vi "main_link.vi"() -> ()   [LabVIEW 2023]
uses:
  <vilib>/Math Plots/3D Math Plots/3D Scatter/3D Scatter XCtrl/3D Scatter.xctl
  HoloTrackerLib/holoTracker.lvlib
  subVis/referencesLINKBtns.ctl
  HoloTrackerLib/dataLink.ctl
  <vilib>/Utility/miscctls.llb/LVMinMaxIncTypeDef.ctl
  subVis/defValuesLink.ctl
  <vilib>/Math Plots/3D Math Plots/3D Scatter/3D Scatter Datatype/3D Scatter Datatype.lvclass
  <vilib>/Math Plots/3D Math Plots/3D Scatter/3D Scatter Datatype/Public/Plot Helper (Vector).vi
  <vilib>/Python/Open Venv Python Session.vi
panel:
  out "Status":string
  in  "Tab Control":enum32{"PATH", "ACTIONS"}(tab)=enum."ACTIONS"
  in  "HoloPath":path caption="feature localisation file path"
  in  "PythonVer":string="3.10" caption="Python version"
  in  "Python/Environnement\npath":path
  in  "step":u16 max=1001 step=1
  in  "history length":u16 max=1001 step=1
  in  "min length":i32
  in  "searchRange":T1={"x_range(m)"=1e-06, "y_range(m)"=1e-06, "z__range(m)"=1e-06}
  in  "memory":i32
  in  "Feature hologram":u16 max=1001 step=1
  in  "SAVE":bool
  out "Total trajectories":u16=95 max=200
  in  "trajectory":u16 max=0
  in  "LINK":bool
  in  "OpenFile":bool
  in  "EXIT":bool
  out "Total holograms":u16=95 max=200
  in  "Play":bool
  in  "CancelPlay":bool
  out "3D Scatter":refnum<class "3D Plot Datatype.lvclass">[](xcontrol)
  # "Link parameters"
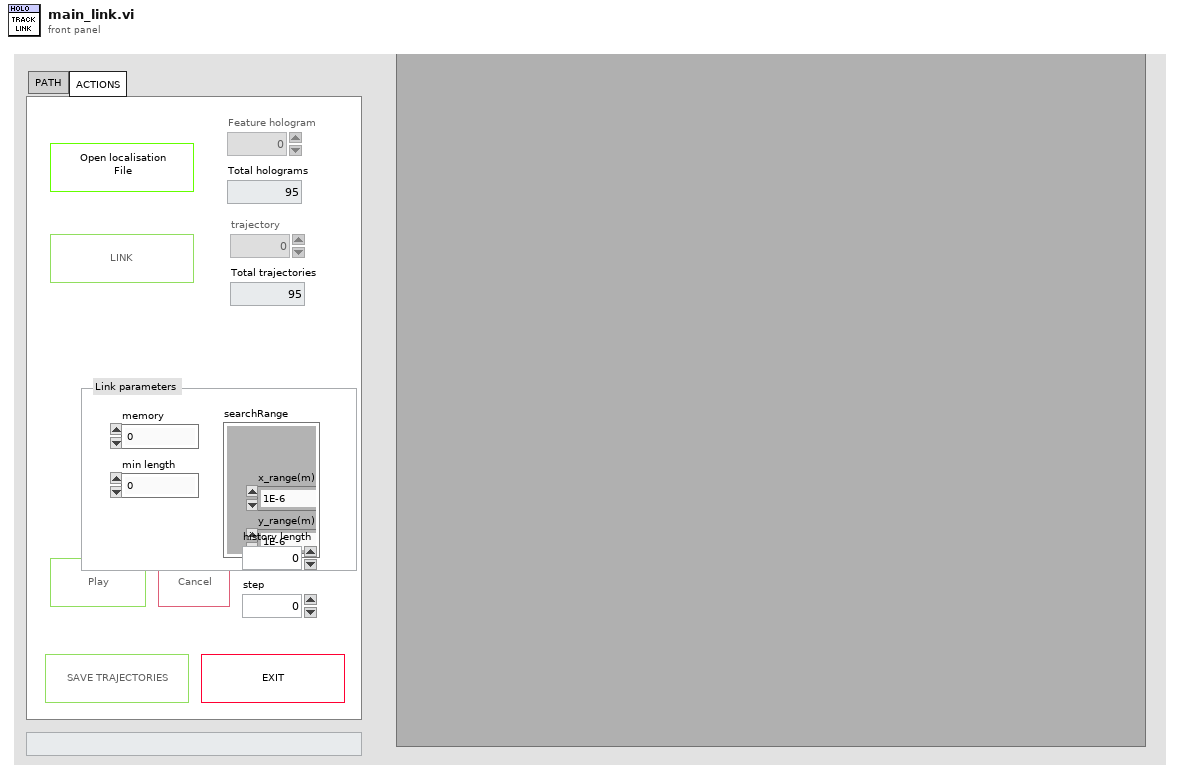
[diagram p1: front panel]
types:
  T1 = cluster{"x_range(m)":dbl, "y_range(m)":dbl, "z__range(m)":dbl}
  T2 = typedef "referencesLINKBtns.ctl" = cluster{"PythonVer":refnum<vi>, "Python/Environnement\npath":refnum<vi>, "HoloPath":refnum<vi>, "HoloDir":refnum<vi>, "Holo parameters":refnum<vi>, "Remove mean Hologram":refnum<vi>, "propagation":refnum<vi>, "Fourier BP filter (pix)":refnum<vi>, "Focus":refnum<vi>, "Batch thresold ":refnum<vi>, "CCL parameters":refnum<vi>, "testMode":refnum<vi>, "exitTestMode":refnum<vi>, "BATCH":refnum<vi>, "CANCEL_BATCH":refnum<vi>, "EXIT":refnum<vi>, "Plane number":refnum<vi>, "Display":refnum<vi>}
  T3 = enum8{"Enabled", "Disabled", "Disabled and Grayed Out"}
  T4 = typedef "dataLink.ctl" = cluster{"PythonSession":refnum<k35>, "Localisations":sgl[][]}
  T5 = enum16{"SESSION CLOSED", "WAIT", "TEST WAIT", "TEST IN PROGESS", "BATCH IN PROGRESS"}
  T6 = typedef "LVMinMaxIncTypeDef.ctl" = cluster{"Minimum":dbl, "Maximum":dbl, "Increment":dbl}
  T7 = cluster{"frame_max":i32, "AllTrajectories":dbl[][]}
  T8 = typedef "defValuesLink.ctl" = cluster{"PythonVer":string, "Python/Environnement\npath":path, "HoloPath":path, "memory":i32, "min length":i32, "searchRange":cluster{"x_range(m)":dbl, "y_range(m)":dbl, "z__range(m)":dbl}}
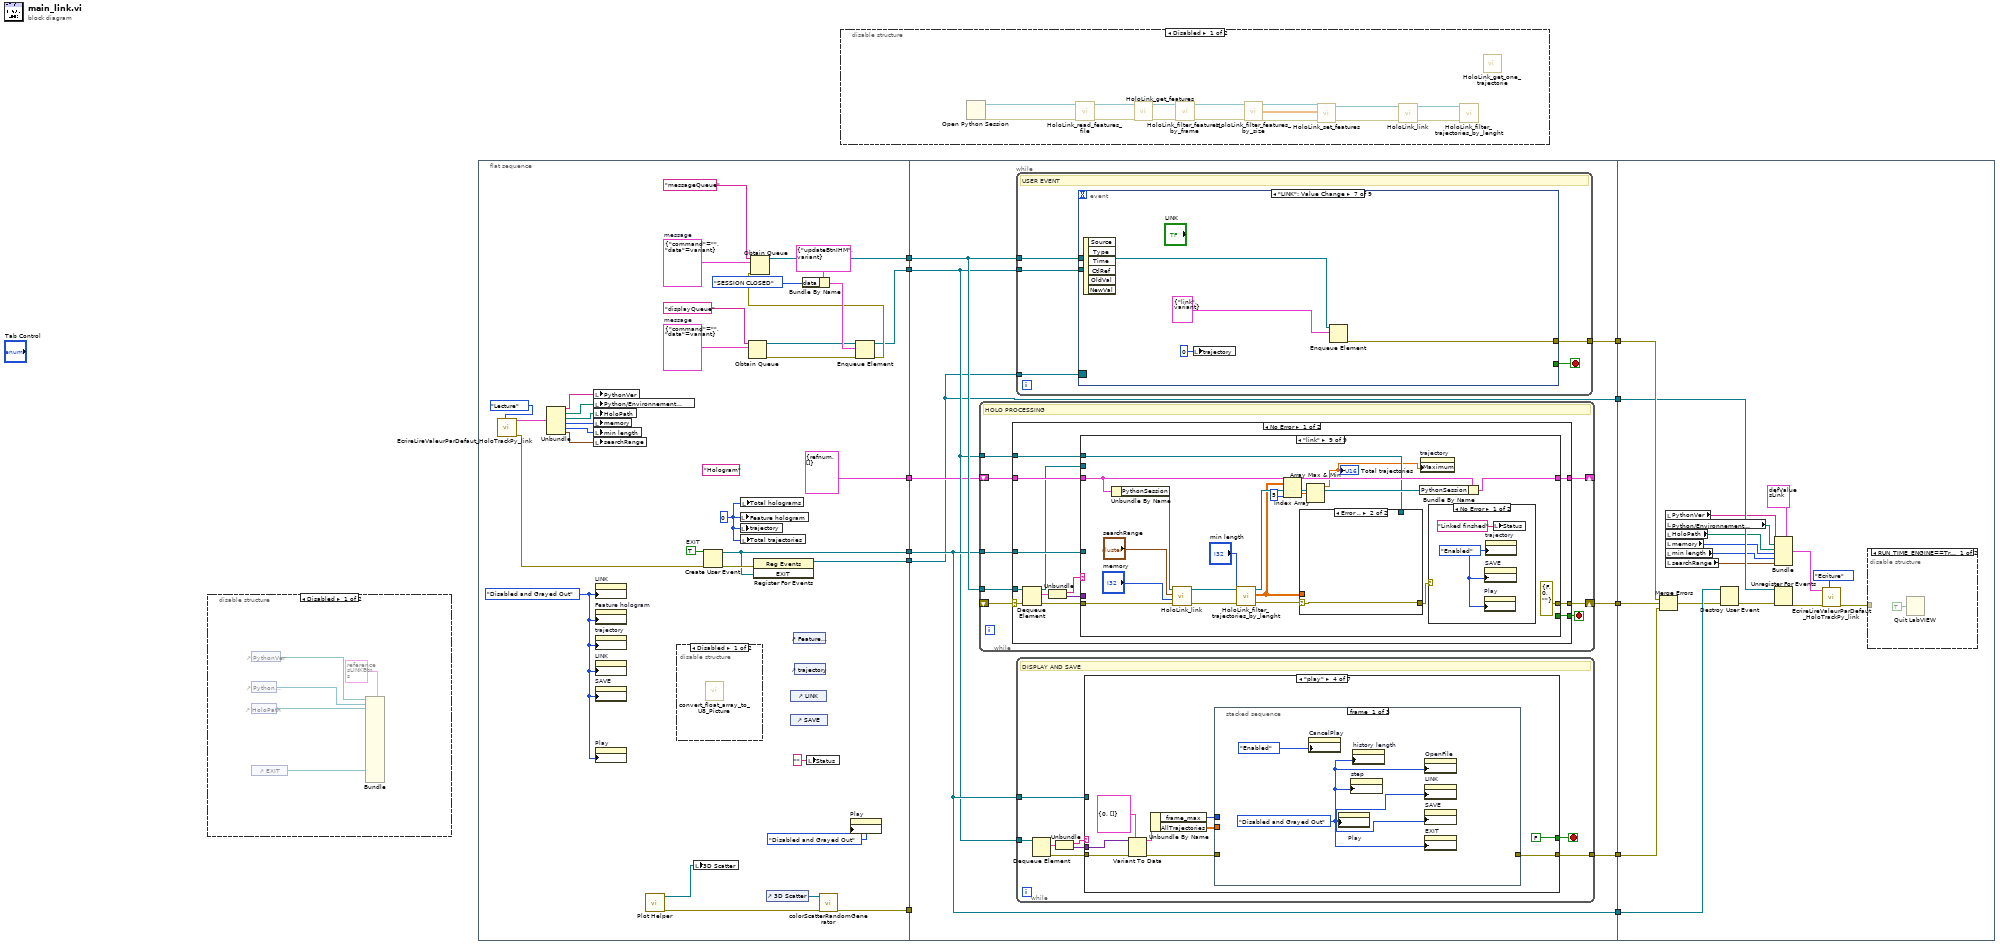
[diagram p0: block diagram]
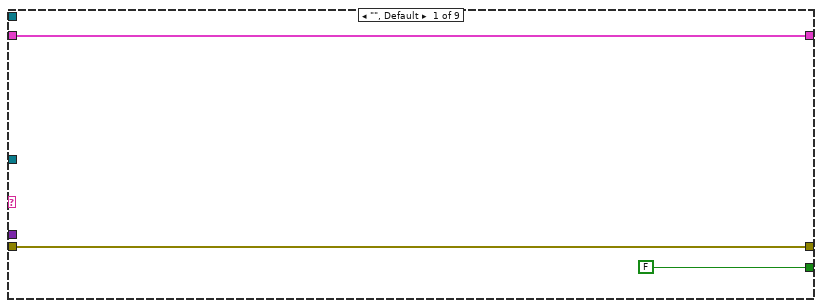
[diagram p5: hidden frame]
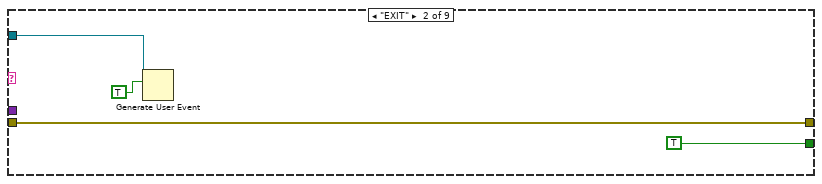
[diagram p6: hidden frame]
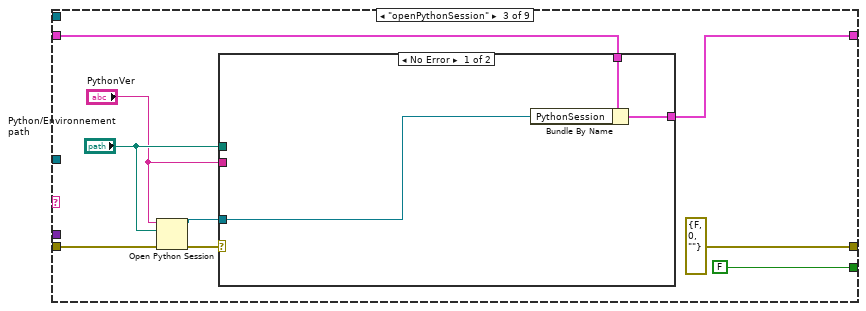
[diagram p7: hidden frame]
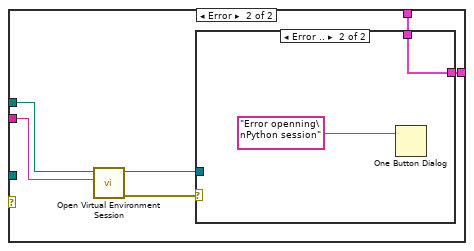
[diagram p8: hidden frame]
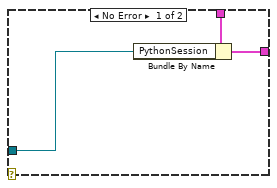
[diagram p9: hidden frame]
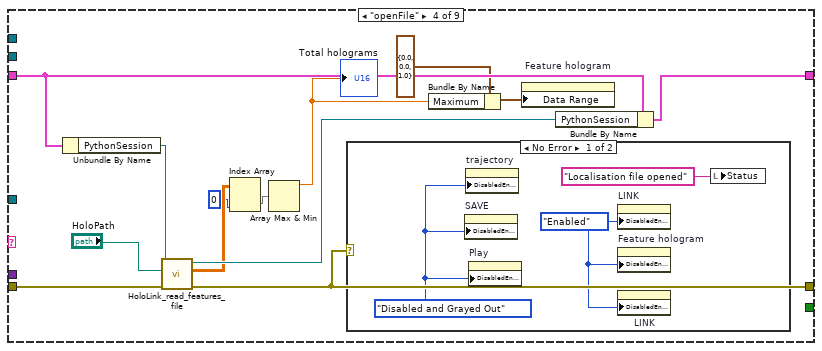
[diagram p10: hidden frame]
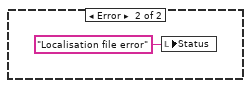
[diagram p11: hidden frame]
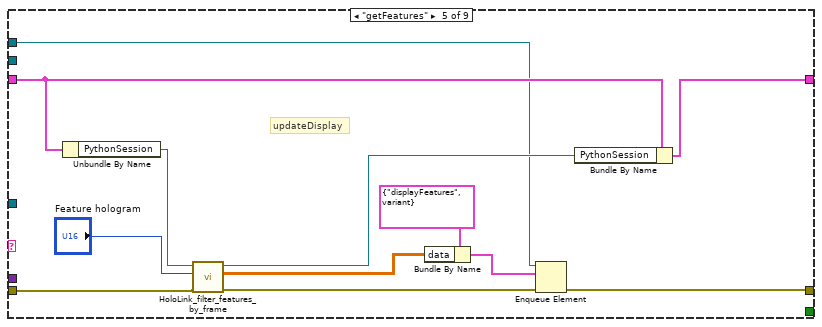
[diagram p12: hidden frame]
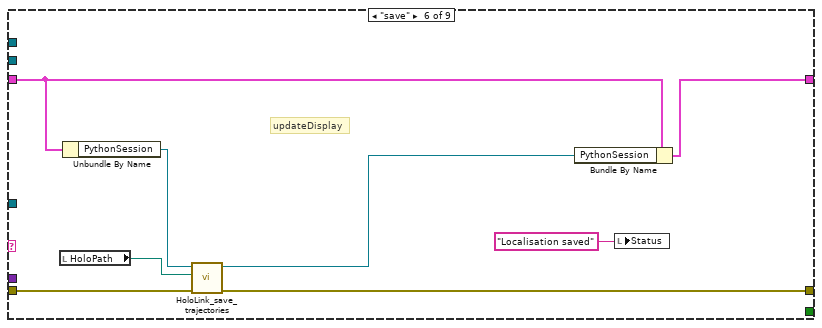
[diagram p13: hidden frame]
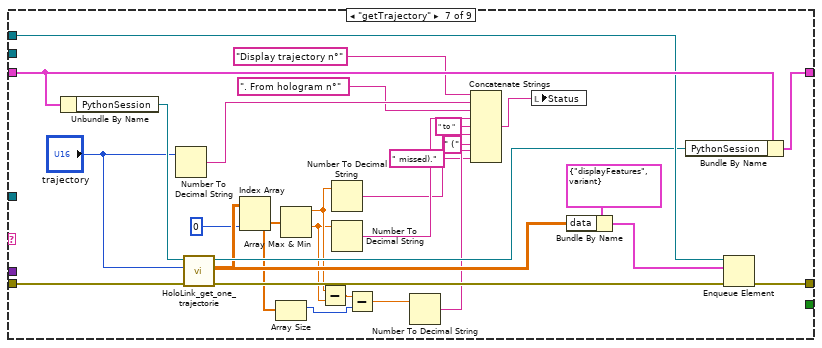
[diagram p14: hidden frame]
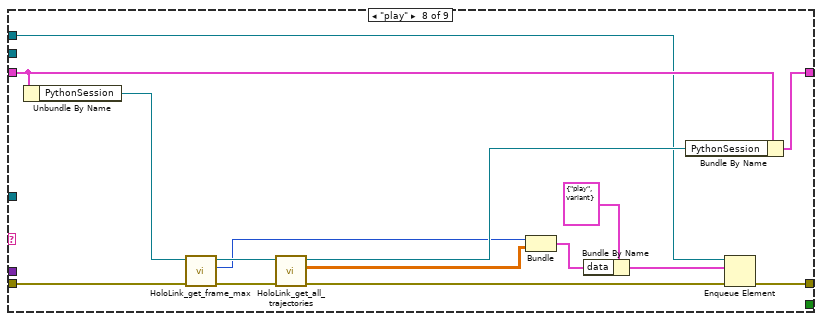
[diagram p15: hidden frame]
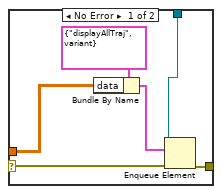
[diagram p16: hidden frame]
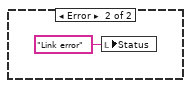
[diagram p17: hidden frame]
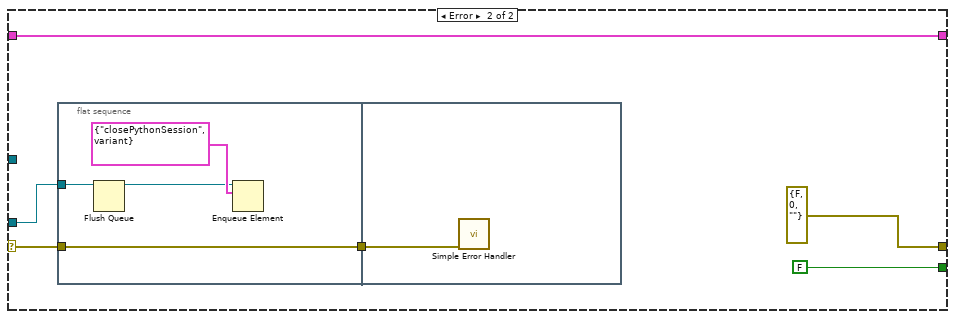
[diagram p18: hidden frame]
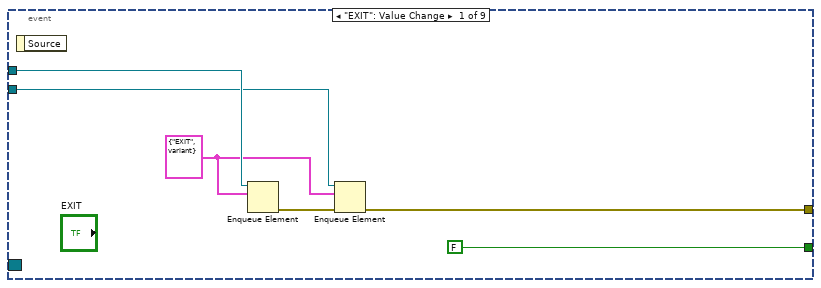
[diagram p19: hidden frame]
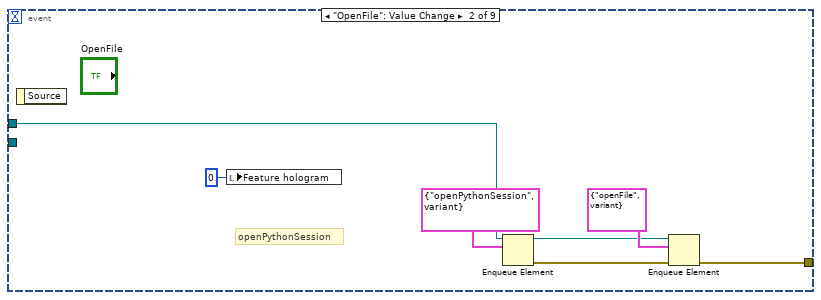
[diagram p20: hidden frame]
diagram:
  n1 = disable-structure shown="Disabled" {
    frame Disabled {
      n2 = control-ref of="EXIT"() -> (w15:refnum<vi>)
      n3 = control-ref of="PythonVer"() -> (w13:refnum<vi>)
      n4 = control-ref of="Python/Environnement\npath"() -> (w14:refnum<vi>)
      n5 = control-ref of="HoloPath"() -> (w16:refnum<vi>)
      n6 = Bundle(cluster=T2 {"PythonVer"=refnum, "Python/Environnement\npath"=refnum, "HoloPath"=refnum, "HoloDir"=refnum, "Holo parameters"=refnum, "Remove mean Hologram"=refnum, "propagation"=refnum, "Fourier BP filter (pix)"=refnum, "Focus"=refnum, "Batch thresold "=refnum, "CCL parameters"=refnum, "testMode"=refnum, "exitTestMode"=refnum, "BATCH"=refnum, "CANCEL_BATCH"=refnum, "EXIT"=refnum, "Plane number"=refnum, "Display"=refnum} ("References"), "PythonVer"=w13, "Python/Environnement\npath"=w14, "HoloPath"=w16, "EXIT"=w15) -> ()  [unwired: 14 in, 1 out]
    }
    frame Enabled {
    }
  }
  n7 = flat-sequence {
    tunnel: [w46] -> w11
    tunnel: [w45] -> w10
    tunnel: [w35] -> w9
    tunnel: [w41] -> w4
    tunnel: [T4 {"PythonSession"=refnum, "Localisations"=[]} ("DatasOUT")] -> w3
    tunnel: [w20] -> w1
    tunnel: w11 -> [w56]
    tunnel: w10 -> [w51]
    tunnel: w9 -> [w55]
    tunnel: [w56] -> w8
    tunnel: [w57] -> w7
    tunnel: [w54] -> w6
    tunnel: [w53] -> w5
    tunnel: w4 -> [w58]
    tunnel: w3 -> [w52]
    tunnel: [w51] -> w2
    tunnel: w1 -> [_]
    tunnel: w8 -> [w395]
    tunnel: w7 -> [w392]
    tunnel: w6 -> [w394]
    tunnel: w5 -> [w393]
    tunnel: w2 -> [w390]
    frame #0 {
      w22 = T3."Disabled and Grayed Out" ("Disabled")
      w32 = u16 0 ("Feature hologram")
      (unwired) "Hologram" ("Label.Text")
      w44 = cluster{"command":string, "data":variant} {"command"="", "data"=variant}  # message
      w48 = TRUE  # EXIT
      w49 = cluster{"command":string, "data":variant} {"command"="", "data"=variant}  # message
      n8 = call "EcrireLireValeurParDefaut_HoloTrackPy_link.vi"("Lecture/Ecriture"=enum32{"Lecture", "Ecriture"}."Lecture") -> ("error out"=w23:errorcluster, "DefValueLinkOUT"=w25:T8)  [unwired: 7 in, 2 out]
      n9 = Unbundle(w25) -> ("PythonVer"=w26:string, "Python/Environnement\npath"=w27:path, "HoloPath"=w28:path, "memory"=w29:i32, "min length"=w30:i32, "searchRange"=w31:T1)
      n10 = local write "PythonVer"(w26) -> ()
      n11 = local write "Python/Environnement\npath"(w27) -> ()
      n12 = local write "HoloPath"(w28) -> ()
      n13 = local write "memory"(w29) -> ()
      n14 = local write "min length"(w30) -> ()
      n15 = local write "searchRange"(w31) -> ()
      n16 = property on="LINK" class="Bool"("DisabledEnum"=w22) -> ()  [unwired: 2 in, 2 out]
      n17 = property on="Feature hologram" class="DigNum (strict)"("DisabledEnum"=w22) -> ()  [unwired: 2 in, 2 out]
      n18 = property on="trajectory" class="DigNum (strict)"("DisabledEnum"=w22) -> ()  [unwired: 2 in, 2 out]
      n19 = property on="LINK" class="Bool"("DisabledEnum"=w22) -> ()  [unwired: 2 in, 2 out]
      n20 = property on="SAVE" class="Bool"("DisabledEnum"=w22) -> ()  [unwired: 2 in, 2 out]
      n21 = property on="Play" class="Bool"("DisabledEnum"=w22) -> ()  [unwired: 2 in, 2 out]
      n22 = call-poly <vilib>:"Plot Helper.vi"() -> ("error out"=w18:errorcluster, "3D Plot lvclass Array out"=w19:refnum<class "3D Plot Datatype.lvclass">[])  [unwired: 6 in, 4 out]
      n23 = disable-structure shown="Disabled" {
        frame Disabled {
          n24 = call "convert_float_array_to_U8_Picture.vi"() -> ()  [unwired: 10 in, 2 out]
        }
        frame Enabled {
        }
      }
      n25 = local write "3D Scatter"(w19) -> ()
      n26 = Create User Event(user event datatype=w48, error in=w23) -> (user event=w46:refnum<user-event>, error out=w47:errorcluster)
      n27 = local write "Feature hologram"(w32) -> ()
      n28 = local write "trajectory"(w32) -> ()
      n29 = local write "Total holograms"(w32) -> ()
      n30 = local write "Total trajectories"(w32) -> ()
      n31 = Obtain Queue(name (unnamed)="displayQueue", element data type=w44) -> (queue out=w38:refnum<queue>, error out=w37:errorcluster)  [unwired: 3 in, 1 out]
      n32 = register-events(error in=w47, w46) -> (reference out=w45:refnum<event-registration>)  [unwired: 1 in, 1 out]
      n33 = control-ref of="3D Scatter"() -> (w21:refnum<vi>)
      n34 = control-ref of="LINK"() -> ()  [unwired: 1 out]
      n35 = control-ref of="SAVE"() -> ()  [unwired: 1 out]
      n36 = control-ref of="Feature hologram"() -> ()  [unwired: 1 out]
      n37 = control-ref of="trajectory"() -> ()  [unwired: 1 out]
      n38 = Bundle By Name(cluster=cluster{"command":string, "data":variant} {"command"="updateBtnIHM", "data"=variant} ("element"), "data"=T5."SESSION CLOSED" ("State")) -> (w39:cluster{"command":string, "data":variant})
      n39 = local write "Status"("" ("Status")) -> ()
      n40 = call "colorScatterRandomGenerator.vi"("error in"=w18, "Control in"=w21) -> ("error out"=w20:errorcluster)  [unwired: 9 in]
      n41 = property on="Play" class="Bool"("DisabledEnum"=T3."Disabled and Grayed Out" ("Disabled")) -> ()  [unwired: 2 in, 2 out]
      n42 = Enqueue Element(queue=w38, element=w39, error in (no error)=w37) -> (queue out=w35:refnum<queue>, error out=w36:errorcluster)  [unwired: 1 in, 1 out]
      n43 = Obtain Queue(name (unnamed)="messageQueue", element data type=w49, error in (no error)=w36) -> (queue out=w41:refnum<queue>)  [unwired: 2 in, 2 out]
    }
    frame #1 {
      n44 = while {
        tunnel: w58 -> [w66]
        tunnel: w56 -> [w64]
        shift-right: [w62] -> _
        shift-left: w52 -> [w63]
        tunnel: w55 -> [w61]
        shift-right: [w60] -> w53
        shift-left: _ -> [w59]
        stop <- w65 stop-if-true
        # "HOLO PROCESSING"
        n45 = case shown="No Error" w59 {
          selector: w59 -> [w69 w223]
          tunnel: w66 -> [w79 w224]
          tunnel: [w74 FALSE] -> w65
          tunnel: w64 -> [w73 _]
          tunnel: w63 -> [w72 w219]
          tunnel: [w67 w219] -> w62
          tunnel: w61 -> [w71 _]
          tunnel: [w68 errorcluster {"status"=FALSE, "code"=0, "source"=""} ("error out")] -> w60
          frame No Error {
            n46 = Dequeue Element(queue=w79, error in (no error)=w69) -> (queue out=w70:refnum<queue>, element=w77:cluster{"command":string, "data":variant}, error out=w78:errorcluster)  [unwired: 1 in, 1 out]
            n47 = Unbundle(w77) -> ("command"=w76:string, "data"=w75:variant)
            n48 = case shown="\"link\"" w76 {
              tunnel: w78 -> [w80 w85 w94 w122 w136 w144 w169 w187 w206]
              tunnel: w75 -> [_ _ _ _ _ _ _ _ _]
              tunnel: [FALSE TRUE FALSE _ _ _ _ _ _] -> w74
              tunnel: w73 -> [_ w83 _ _ _ _ _ _ _]
              tunnel: w72 -> [w81 _ w91 w119 w138 w146 w175 w190 w208]
              tunnel: [w81 _ w90 w117 w137 w145 w174 w189 w207] -> w67
              tunnel: w71 -> [_ _ _ _ w130 _ w172 w176 w197]
              tunnel: [w80 w85 errorcluster {"status"=FALSE, "code"=0, "source"=""} ("error out") w116 w131 w141 w173 w181 errorcluster {"status"=FALSE, "code"=0, "source"=""} ("error out")] -> w68
              tunnel: w70 -> [_ _ _ _ _ _ _ _ _]
              frame "", Default {
              }
              frame "EXIT" {
                n49 = Generate User Event(user event=w83, event data cluster=TRUE ("event data")) -> ()  [unwired: 2 in, 2 out]
              }
              frame "openPythonSession" {
                n50 = Open Python Session(python version="PythonVer", python path="Python/Environnement\npath", 3:w94) -> (session out=w88:refnum<k35>, error out=w93:errorcluster)
                n51 = case shown="No Error" w93 {
                  tunnel: "Python/Environnement\npath" -> [_ w104]
                  tunnel: "PythonVer" -> [_ w103]
                  tunnel: w91 -> [w98 w101]
                  tunnel: [w97 w100] -> w90
                  tunnel: w88 -> [w96 _]
                  frame No Error {
                    n52 = Bundle By Name(cluster=w98, "PythonSession"=w96) -> (w97:T4)
                  }
                  frame Error {
                    n53 = call-poly <vilib>:"Open Virtual Environment Session.vi"("Python version"=w103, "Env path"=w104) -> ("error out"=w102:errorcluster, "session out"=w99:refnum<k35>)  [unwired: 8 in]
                    n54 = case shown="Error .." w102 {
                      tunnel: w101 -> [w107 w108]
                      tunnel: [w106 w108] -> w100
                      tunnel: w99 -> [w105 _]
                      frame No Error {
                        n55 = Bundle By Name(cluster=w107, "PythonSession"=w105) -> (w106:T4)
                      }
                      frame Error {
                        n56 = One Button Dialog(message="Error openning\nPython session") -> ()  [unwired: 1 in, 1 out]
                      }
                    }
                  }
                }
              }
              frame "openFile" {
                n57 = Unbundle By Name(w119) -> ("PythonSession"=w121:refnum<k35>)
                n58 = call "HoloLink_read_features_file.vi"("error in (no error)"=w122, "holo Feature file"="HoloPath", "session in"=w121) -> ("error out"=w116:errorcluster, "localisations"=w115:dbl[][], "Refnum out"=w118:refnum<k35>)  [unwired: 6 in]
                n59 = Index Array(array=w115, index (col)=0 ("index (row)")) -> (element=w114:dbl[])  [unwired: 1 in]
                n60 = Array Max & Min(array=w114) -> (max value=w111:dbl)  [unwired: 3 out]
                "Total holograms" <- w111
                n61 = case shown="No Error" w116 {
                  frame No Error {
                    w123 = T3."Disabled and Grayed Out" ("Disabled")
                    w124 = T3."Enabled" ("Disabled")
                    n62 = property on="SAVE" class="Bool"("DisabledEnum"=w123) -> ()  [unwired: 2 in, 2 out]
                    n63 = property on="trajectory" class="DigNum (strict)"("DisabledEnum"=w123) -> ()  [unwired: 2 in, 2 out]
                    n64 = property on="Play" class="Bool"("DisabledEnum"=w123) -> ()  [unwired: 2 in, 2 out]
                    n65 = property on="LINK" class="Bool"("DisabledEnum"=w124) -> ()  [unwired: 2 in, 2 out]
                    n66 = property on="Feature hologram" class="DigNum (strict)"("DisabledEnum"=w124) -> ()  [unwired: 2 in, 2 out]
                    n67 = property on="LINK" class="Bool"("DisabledEnum"=w124) -> ()  [unwired: 2 in, 2 out]
                    n68 = local write "Status"("Localisation file opened" ("Status")) -> ()
                  }
                  frame Error {
                    n69 = local write "Status"("Localisation file error" ("Status")) -> ()
                  }
                }
                n70 = Bundle By Name(cluster=T6 {"Minimum"=0.0, "Maximum"=0.0, "Increment"=1.0} ("Data Entry Limits"), "Maximum"=w111) -> (w112:T6)
                n71 = property on="Feature hologram" class="DigNum (strict)"("Data Range"=w112) -> ()  [unwired: 2 in, 2 out]
                n72 = Bundle By Name(cluster=w119, "PythonSession"=w118) -> (w117:T4)
              }
              frame "getFeatures" {
                # "updateDisplay"
                n73 = Unbundle By Name(w138) -> ("PythonSession"=w135:refnum<k35>)
                n74 = call "HoloLink_filter_features_by_frame.vi"("error in (no error)"=w136, "Frame"="Feature hologram", "session in"=w135) -> ("error out"=w132:errorcluster, "return value"=w127:dbl[][], "Refnum out"=w134:refnum<k35>)  [unwired: 6 in]
                n75 = Bundle By Name(cluster=cluster{"command":string, "data":variant} {"command"="displayFeatures", "data"=variant} ("element"), "data"=w127) -> (w128:cluster{"command":string, "data":variant})
                n76 = Enqueue Element(queue=w130, element=w128, error in (no error)=w132) -> (error out=w131:errorcluster)  [unwired: 1 in, 2 out]
                n77 = Bundle By Name(cluster=w138, "PythonSession"=w134) -> (w137:T4)
              }
              frame "save" {
                # "updateDisplay"
                n78 = local read "HoloPath"() -> (w139:path)
                n79 = Unbundle By Name(w146) -> ("PythonSession"=w143:refnum<k35>)
                n80 = call "HoloLink_save_trajectories.vi"("error in (no error)"=w144, "holo Feature file"=w139, "session in"=w143) -> ("error out"=w141:errorcluster, "Refnum out"=w142:refnum<k35>)  [unwired: 7 in]
                n81 = Bundle By Name(cluster=w146, "PythonSession"=w142) -> (w145:T4)
                n82 = local write "Status"("Localisation saved" ("Status")) -> ()
              }
              frame "getTrajectory" {
                n83 = Unbundle By Name(w175) -> ("PythonSession"=w167:refnum<k35>)
                n84 = Number To Decimal String(number="trajectory") -> (decimal integer string=w163:string)  [unwired: 1 in]
                n85 = call "HoloLink_get_one_trajectorie.vi"("error in (no error)"=w169, "feature_number"="trajectory", "session in"=w167) -> ("error out"=w168:errorcluster, "trajectorie"=w162:dbl[][], "Refnum out"=w166:refnum<k35>)  [unwired: 6 in]
                n86 = Index Array(array=w162, index (col)=0 ("disabled index (col)")) -> (element=w154:dbl[])  [unwired: 1 in]
                n87 = Array Size(array=w154) -> (size(s)=w149:i32)
                n88 = Array Max & Min(array=w154) -> (max value=w152:dbl, min value=w151:dbl)  [unwired: 2 out]
                n89 = Subtract(x=w152, y=w151) -> (x-y=w150:dbl)
                n90 = Number To Decimal String(number=w152) -> (decimal integer string=w155:string)  [unwired: 1 in]
                n91 = Number To Decimal String(number=w151) -> (decimal integer string=w156:string)  [unwired: 1 in]
                n92 = Subtract(x=w150, y=w149) -> (x-y=w148:dbl)
                n93 = Number To Decimal String(number=w148) -> (decimal integer string=w153:string)  [unwired: 1 in]
                n94 = Concatenate Strings("Display trajectory n°" ("Status"), w163, ". From hologram n°" ("string"), w156, " to " ("string"), w155, " (" ("string"), w153, " missed)." ("string")) -> (w157:string)
                n95 = local write "Status"(w157) -> ()
                n96 = Bundle By Name(cluster=cluster{"command":string, "data":variant} {"command"="displayFeatures", "data"=variant} ("element"), "data"=w162) -> (w170:cluster{"command":string, "data":variant})
                n97 = Bundle By Name(cluster=w175, "PythonSession"=w166) -> (w174:T4)
                n98 = Enqueue Element(queue=w172, element=w170, error in (no error)=w168) -> (error out=w173:errorcluster)  [unwired: 1 in, 2 out]
              }
              frame "play" {
                n99 = Unbundle By Name(w190) -> ("PythonSession"=w188:refnum<k35>)
                n100 = call "HoloLink_get_frame_max.vi"("error in (no error)"=w187, "session in"=w188) -> ("error out"=w184:errorcluster, "frame_max"=w178:i32, "Refnum out"=w183:refnum<k35>)  [unwired: 7 in]
                n101 = call "HoloLink_get_all_trajectories.vi"("error in (no error)"=w184, "session in"=w183) -> ("error out"=w182:errorcluster, "AllTrajectories"=w179:dbl[][], "Refnum out"=w180:refnum<k35>)  [unwired: 7 in]
                n102 = Bundle("frame_max"=w178, "AllTrajectories"=w179) -> (w177:T7)  [unwired: 1 in]
                n103 = Bundle By Name(cluster=cluster{"command":string, "data":variant} {"command"="play", "data"=variant} ("element"), "data"=w177) -> (w186:cluster{"command":string, "data":variant})
                n104 = Bundle By Name(cluster=w190, "PythonSession"=w180) -> (w189:T4)
                n105 = Enqueue Element(queue=w176, element=w186, error in (no error)=w182) -> (error out=w181:errorcluster)  [unwired: 1 in, 2 out]
              }
              frame "link" {
                n106 = Unbundle By Name(w208) -> ("PythonSession"=w205:refnum<k35>)
                n107 = call "HoloLink_link.vi"("error in (no error)"=w206, "memory"="memory", "searchRange"="searchRange", "session in"=w205) -> ("error out"=w202:errorcluster, "Refnum out"=w201:refnum<k35>)  [unwired: 5 in, 1 out]
                n108 = call "HoloLink_filter_trajectories_by_lenght.vi"("error in (no error)"=w202, "minLenght"="min length", "session in"=w201) -> ("error out"=w192:errorcluster, "return value"=w195:dbl[][], "Refnum out"=w200:refnum<k35>)  [unwired: 6 in]
                n109 = Index Array(array=w195, index (col)=5 ("index (row)")) -> (element=w196:dbl[])  [unwired: 1 in]
                n110 = case shown="Error .." w192 {
                  selector: w192 -> [w209 w215]
                  tunnel: [w212 w215] -> w198
                  tunnel: w197 -> [w211 _]
                  tunnel: w195 -> [w210 _]
                  frame No Error {
                    n111 = Bundle By Name(cluster=cluster{"command":string, "data":variant} {"command"="displayAllTraj", "data"=variant} ("element"), "data"=w210) -> (w213:cluster{"command":string, "data":variant})
                    n112 = Enqueue Element(queue=w211, element=w213, error in (no error)=w209) -> (error out=w212:errorcluster)  [unwired: 1 in, 2 out]
                  }
                  frame Error {
                  }
                }
                n113 = Array Max & Min(array=w196) -> (max value=w194:dbl)  [unwired: 3 out]
                "Total trajectories" <- w194
                n114 = Bundle By Name(cluster=w208, "PythonSession"=w200) -> (w207:T4)
                n115 = property on="trajectory" class="DigNum (strict)"("Maximum"=w194) -> ()  [unwired: 2 in, 2 out]
                n116 = case shown="No Error" w198 {
                  frame No Error {
                    w216 = T3."Enabled" ("Disabled")
                    n117 = property on="Play" class="Bool"("DisabledEnum"=w216) -> ()  [unwired: 2 in, 2 out]
                    n118 = property on="SAVE" class="Bool"("DisabledEnum"=w216) -> ()  [unwired: 2 in, 2 out]
                    n119 = property on="trajectory" class="DigNum (strict)"("DisabledEnum"=w216) -> ()  [unwired: 2 in, 2 out]
                    n120 = local write "Status"("Linked finshed" ("Status")) -> ()
                  }
                  frame Error {
                    n121 = local write "Status"("Link error" ("Status")) -> ()
                  }
                }
              }
            }
          }
          frame Error {
            n122 = flat-sequence {
              tunnel: w224 -> [w226]
              tunnel: w223 -> [w227]
              tunnel: [w227] -> w222
              tunnel: w222 -> [w229]
              frame #0 {
                n123 = Flush Queue(queue=w226) -> (queue out=w225:refnum<queue>)  [unwired: 1 in, 2 out]
                n124 = Enqueue Element(queue=w225, element=cluster{"command":string, "data":variant} {"command"="closePythonSession", "data"=variant}) -> ()  [unwired: 2 in, 3 out]
              }
              frame #1 {
                n125 = call <vilib>:"Simple Error Handler.vi"("error in (no error)"=w229) -> ()  [unwired: 4 in, 5 out]
              }
            }
          }
        }
      }
      n126 = while {
        tunnel: w58 -> [w233]
        tunnel: w51 -> [w232]
        tunnel: [w231] -> w57
        tunnel: w55 -> [w230]
        stop <- w234 stop-if-true
        # "USER EVENT"
        n127 = event shown="[6] \"LINK\": Value Change" {
          selector: w232 -> [_ _ _ _ _ _ _ _ _]
          dyn-events: _ -> [_ _ _ _ _ _ _ _ _]
          timeout: _ -> [_ _ _ _ _ _ _ _ _]
          tunnel: [FALSE _ _ _ _ _ _ FALSE TRUE] -> w234
          tunnel: w233 -> [w239 w244 w250 w253 w256 w259 w263 w270 _]
          tunnel: [w235 w246 w248 w251 w254 w257 w261 w269 _] -> w231
          tunnel: w230 -> [w237 _ _ _ _ _ _ w264 _]
          event "EXIT": Value Change {
            w238 = cluster{"command":string, "data":variant} {"command"="EXIT", "data"=variant} ("element")
            n128 = event-data() -> ()  [unwired: 1 in, 1 out]
            n129 = Enqueue Element(queue=w239, element=w238) -> (error out=w236:errorcluster)  [unwired: 2 in, 2 out]
            n130 = Enqueue Element(queue=w237, element=w238, error in (no error)=w236) -> (error out=w235:errorcluster)  [unwired: 1 in, 2 out]
          }
          event "OpenFile": Value Change {
            # "openPythonSession"
            n131 = event-data() -> ()  [unwired: 1 in, 1 out]
            n132 = local write "Feature hologram"(u16 0 ("Feature hologram")) -> ()
            n133 = Enqueue Element(queue=w244, element=cluster{"command":string, "data":variant} {"command"="openPythonSession", "data"=variant}) -> (queue out=w243:refnum<queue>, error out=w242:errorcluster)  [unwired: 2 in, 1 out]
            n134 = Enqueue Element(queue=w243, element=cluster{"command":string, "data":variant} {"command"="openFile", "data"=variant}, error in (no error)=w242) -> (error out=w246:errorcluster)  [unwired: 1 in, 2 out]
          }
          event "Feature hologram": Value Change {
            n135 = event-data() -> ()  [unwired: 1 in, 6 out]
            n136 = Enqueue Element(queue=w250, element=cluster{"command":string, "data":variant} {"command"="getFeatures", "data"=variant}) -> (error out=w248:errorcluster)  [unwired: 2 in, 2 out]
          }
          event "Play": Value Change {
            n137 = event-data() -> ()  [unwired: 1 in, 6 out]
            n138 = Enqueue Element(queue=w253, element=cluster{"command":string, "data":variant} {"command"="play", "data"=variant}) -> (error out=w251:errorcluster)  [unwired: 2 in, 2 out]
          }
          event "SAVE": Value Change {
            n139 = event-data() -> ()  [unwired: 1 in, 6 out]
            n140 = Enqueue Element(queue=w256, element=cluster{"command":string, "data":variant} {"command"="save", "data"=variant}) -> (error out=w254:errorcluster)  [unwired: 2 in, 2 out]
          }
          event "trajectory": Value Change {
            n141 = event-data() -> ()  [unwired: 1 in, 6 out]
            n142 = Enqueue Element(queue=w259, element=cluster{"command":string, "data":variant} {"command"="getTrajectory", "data"=variant}) -> (error out=w257:errorcluster)  [unwired: 2 in, 2 out]
          }
          event "LINK": Value Change {
            n143 = event-data() -> ()  [unwired: 1 in, 6 out]
            n144 = local write "trajectory"(u16 0 ("trajectory")) -> ()
            n145 = Enqueue Element(queue=w263, element=cluster{"command":string, "data":variant} {"command"="link", "data"=variant}) -> (error out=w261:errorcluster)  [unwired: 2 in, 2 out]
          }
          event Panel Close? {
            n146 = event-data() -> ()  [unwired: 1 in, 4 out]
            n147 = Two Button Dialog(message="EXIT APPLICATION?", 2:"YES" ("T button name (\"OK\")")) -> (T button?=w266:bool)  [unwired: 1 in]
            n148 = case shown="True" w266 {
              tunnel: w270 -> [_ w277]
              tunnel: [errorcluster {"status"=FALSE, "code"=0, "source"=""} ("error out") w273] -> w269
              tunnel: w264 -> [_ w275]
              frame False {
              }
              frame True {
                w274 = cluster{"command":string, "data":variant} {"command"="EXIT", "data"=variant} ("element")
                n149 = Enqueue Element(queue=w277, element=w274) -> (error out=w276:errorcluster)  [unwired: 2 in, 2 out]
                n150 = Enqueue Element(queue=w275, element=w274, error in (no error)=w276) -> (error out=w273:errorcluster)  [unwired: 1 in, 2 out]
              }
            }
            n151 = event-data("Discard?"=TRUE) -> ()  [unwired: 1 in, 1 out]
          }
          event User Event {
            n152 = event-data() -> ()  [unwired: 1 in, 5 out]
          }
        }
      }
      n153 = while {
        tunnel: w55 -> [w286]
        tunnel: w56 -> [w280]
        tunnel: [w279] -> w54
        stop <- w281 stop-if-true
        # "DISPLAY AND SAVE"
        n154 = Dequeue Element(queue=w286) -> (element=w284:cluster{"command":string, "data":variant}, error out=w285:errorcluster)  [unwired: 2 in, 2 out]
        n155 = Unbundle(w284) -> ("command"=w283:string, "data"=w282:variant)
        n156 = case shown="\"play\"" w283 {
          tunnel: w285 -> [w287 w294 w302 w313 w350 w376 w377]
          tunnel: w282 -> [_ w293 w301 w312 w349 w375 _]
          tunnel: [FALSE FALSE FALSE FALSE FALSE FALSE TRUE] -> w281
          tunnel: w280 -> [_ _ _ _ _ _ _]
          tunnel: [w287 w290 w298 w306 w345 w373 w377] -> w279
          frame "", Default {
          }
          frame "updateStatus" {
            n157 = Variant To Data(error in=w294, type="" ("return value"), Variant=w293) -> (data=→"Status":string, error out=w290:errorcluster)
          }
          frame "displayFeatures" {
            n158 = Variant To Data(error in=w302, type=sgl[][] [] ("y"), Variant=w301) -> (data=w295:sgl[][], error out=w298:errorcluster)
            n159 = Not Equal?(x=w295, y=sgl[][] []) -> (x != y?=w296:bool)
            n160 = case shown="True" w296 {
              tunnel: w295 -> [_ w304]
              frame False {
              }
              frame True {
                n161 = call "setScatterColor.vi"("Features"=w304) -> ("3D Plot lvclass Array out"=→"3D Scatter":refnum<class "3D Plot Datatype.lvclass">[])  [unwired: 10 in]
              }
            }
          }
          frame "play" {
            n162 = Variant To Data(error in=w313, type=T7 {"frame_max"=0, "AllTrajectories"=[]} ("output cluster"), Variant=w312) -> (data=w308:T7, error out=w309:errorcluster)
            n163 = Unbundle By Name(w308) -> ("frame_max"=w305:i32, "AllTrajectories"=w307:dbl[][])
            n164 = stacked-sequence {
              tunnel: w309 -> [_ w323 _]
              tunnel: w307 -> [_ w322 _]
              tunnel: [_ w321 _] -> w306
              tunnel: w305 -> [_ w319 _]
              frame #0 {
                w314 = T3."Disabled and Grayed Out" ("Disabled")
                n165 = property on="CancelPlay" class="Bool"("DisabledEnum"=T3."Enabled" ("Disabled")) -> ()  [unwired: 2 in, 2 out]
                n166 = property on="Play" class="Bool"("DisabledEnum"=w314) -> ()  [unwired: 2 in, 2 out]
                n167 = property on="step" class="DigNum (strict)"("DisabledEnum"=w314) -> ()  [unwired: 2 in, 2 out]
                n168 = property on="history length" class="DigNum (strict)"("DisabledEnum"=w314) -> ()  [unwired: 2 in, 2 out]
                n169 = property on="OpenFile" class="Bool"("DisabledEnum"=w314) -> ()  [unwired: 2 in, 2 out]
                n170 = property on="LINK" class="Bool"("DisabledEnum"=w314) -> ()  [unwired: 2 in, 2 out]
                n171 = property on="SAVE" class="Bool"("DisabledEnum"=w314) -> ()  [unwired: 2 in, 2 out]
                n172 = property on="EXIT" class="Bool"("DisabledEnum"=w314) -> ()  [unwired: 2 in, 2 out]
              }
              frame #1 {
                n173 = Subtract(x=w319, y="history length") -> (x-y=w320:i32)
                n174 = Divide(x=w320, y="step") -> (x/y=w318:dbl)
                n175 = for {
                  N: w318 -> [_]
                  shift-right: [w331] -> w321
                  shift-left: w323 -> [w333]
                  tunnel: w322 -> [w332]
                  tunnel: "step" -> [w330]
                  tunnel: "history length" -> [w329]
                  i -> [w334]
                  stop <- "CancelPlay" stop-if-true
                  n176 = Multiply(x=w334, y=w330) -> (x*y=w325:i32)
                  n177 = Add(x=w325, y=w329) -> (x+y=w324:i32)
                  n178 = Number To Decimal String(number=w324) -> (decimal integer string=w336:string)  [unwired: 1 in]
                  n179 = Number To Decimal String(number=w325) -> (decimal integer string=w339:string)  [unwired: 1 in]
                  n180 = call "filterPortionTrajectories.vi"("error in (no error)"=w333, "ToHoloN°"=w324, "FromHoloN°"=w325, "AllTrajectories in"=w332) -> ("error out"=w331:errorcluster, "AllTrajectories out"=w327:dbl[][])  [unwired: 6 in]
                  n181 = call "setScatterColor.vi"("Features"=w327) -> ("3D Plot lvclass Array out"=w326:refnum<class "3D Plot Datatype.lvclass">[])  [unwired: 10 in]
                  n182 = Concatenate Strings("Display portion from " ("Status"), w339, " to " ("string"), w336, "." ("string")) -> (w337:string)
                  n183 = local write "3D Scatter"(w326) -> ()
                  n184 = local write "Status"(w337) -> ()
                }
              }
              frame #2 {
                w341 = T3."Enabled" ("Disabled")
                n185 = property on="CancelPlay" class="Bool"("DisabledEnum"=T3."Disabled and Grayed Out" ("Disabled")) -> ()  [unwired: 2 in, 2 out]
                n186 = property on="Play" class="Bool"("DisabledEnum"=w341) -> ()  [unwired: 2 in, 2 out]
                n187 = property on="step" class="DigNum (strict)"("DisabledEnum"=w341) -> ()  [unwired: 2 in, 2 out]
                n188 = property on="history length" class="DigNum (strict)"("DisabledEnum"=w341) -> ()  [unwired: 2 in, 2 out]
                n189 = property on="OpenFile" class="Bool"("DisabledEnum"=w341) -> ()  [unwired: 2 in, 2 out]
                n190 = property on="LINK" class="Bool"("DisabledEnum"=w341) -> ()  [unwired: 2 in, 2 out]
                n191 = property on="SAVE" class="Bool"("DisabledEnum"=w341) -> ()  [unwired: 2 in, 2 out]
                n192 = property on="EXIT" class="Bool"("DisabledEnum"=w341) -> ()  [unwired: 2 in, 2 out]
              }
            }
          }
          frame "displayAllTraj" {
            n193 = Variant To Data(error in=w350, type=sgl[][] [] ("y"), Variant=w349) -> (data=w343:sgl[][], error out=w345:errorcluster)
            n194 = Not Equal?(x=w343, y=sgl[][] []) -> (x != y?=w347:bool)
            n195 = case shown="True" w347 {
              tunnel: w343 -> [_ w352]
              frame False {
              }
              frame True {
                w370 = 1000000.0
                n196 = Index Array(array=w352, index (col) #1=1 ("disabled index (col)"), index (col) #2=2 ("index (col)"), index (col) #3=3 ("index (col)")) -> (element #1=w364:sgl[], element #2=w363:sgl[], element #3=w371:sgl[])  [unwired: 3 in]
                n197 = Multiply(x=w364, y=w370) -> (x*y=w366:dbl[])
                n198 = Multiply(x=w363, y=w370) -> (x*y=w362:dbl[])
                n199 = Multiply(x=w371, y=w370) -> (x*y=w361:dbl[])
                n200 = Array Max & Min(array=w366) -> (max value=w358:dbl, min value=w357:dbl)  [unwired: 2 out]
                n201 = Array Max & Min(array=w362) -> (max value=w356:dbl, min value=w355:dbl)  [unwired: 2 out]
                n202 = Array Max & Min(array=w361) -> (max value=w354:dbl, min value=w353:dbl)  [unwired: 2 out]
                n203 = call "setScatterColor.vi"("Features"=w352) -> ("3D Plot lvclass Array out"=w351:refnum<class "3D Plot Datatype.lvclass">[])  [unwired: 10 in]
                n204 = property on="3D Scatter" class="3D Scatter (strict)"("Axis:Active Axis"=enum16{"X-axis", "Y-axis", "Z-axis"}."X-axis", "Axis:Range Maximum"=w358, "Axis:Range Minimum"=w357) -> ()  [unwired: 2 in, 2 out]
                n205 = local write "3D Scatter"(w351) -> ()
                n206 = property on="3D Scatter" class="3D Scatter (strict)"("Axis:Active Axis"=enum16{"X-axis", "Y-axis", "Z-axis"}."Z-axis", "Axis:Range Maximum"=w354, "Axis:Range Minimum"=w353) -> ()  [unwired: 2 in, 2 out]
                n207 = property on="3D Scatter" class="3D Scatter (strict)"("Axis:Active Axis"=enum16{"X-axis", "Y-axis", "Z-axis"}."Y-axis", "Axis:Range Maximum"=w356, "Axis:Range Minimum"=w355) -> ()  [unwired: 2 in, 2 out]
              }
            }
          }
          frame "updateLabelPicture" {
            n208 = Variant To Data(error in=w376, type="label" ("Label.Text"), Variant=w375) -> (error out=w373:errorcluster)  [unwired: 1 out]
          }
          frame "EXIT" {
          }
        }
      }
    }
    frame #2 {
      n209 = Merge Errors(w392, w393, w394) -> (w391:errorcluster)
      n210 = local read "PythonVer"() -> (w384:string)
      n211 = local read "Python/Environnement\npath"() -> (w385:path)
      n212 = local read "HoloPath"() -> (w386:path)
      n213 = local read "memory"() -> (w387:i32)
      n214 = local read "min length"() -> (w388:i32)
      n215 = local read "searchRange"() -> (w389:T1)
      n216 = Destroy User Event(user event=w395, error in=w391) -> (error out=w396:errorcluster)
      n217 = Bundle(cluster=T8 {"PythonVer"="", "Python/Environnement\npath"=path "", "HoloPath"=path "", "memory"=0, "min length"=0, "searchRange"={"x_range(m)"=0.0, "y_range(m)"=0.0, "z__range(m)"=0.0}} ("DefValueLink"), "PythonVer"=w384, "Python/Environnement\npath"=w385, "HoloPath"=w386, "memory"=w387, "min length"=w388, "searchRange"=w389) -> (w379:T8)
      n218 = Unregister For Events(event registration refnum=w390, error in=w396) -> (error out=w382:errorcluster)
      n219 = call "EcrireLireValeurParDefaut_HoloTrackPy_link.vi"("Lecture/Ecriture"=enum32{"Lecture", "Ecriture"}."Ecriture", "error in (no error)"=w382, "DefValueLinkIN"=w379) -> ("error out"=w381:errorcluster)  [unwired: 5 in, 3 out]
      n220 = disable-structure shown="RUN_TIME_ENGINE==True" {
        disable-tunnel: w381 -> [_ _]
        frame condition #0 {
          n221 = Quit LabVIEW(quit? (T)=TRUE) -> ()
        }
        frame condition #1 (active) {
        }
      }
    }
  }
  n222 = disable-structure shown="Disabled" {
    frame Disabled {
      n223 = Open Python Session() -> (session out=w418:refnum<k35>, error out=w417:errorcluster)  [unwired: 3 in]
      n224 = call "HoloLink_read_features_file.vi"("error in (no error)"=w417, "session in"=w418) -> ("error out"=w415:errorcluster, "localisations"=w407:dbl[][], "Refnum out"=w414:refnum<k35>, "holo Feature file"=w416:path)  [unwired: 6 in]
      n225 = call "HoloLink_get_features.vi"("error in (no error)"=w415, "session in"=w414) -> ("error out"=w412:errorcluster, "Refnum out"=w413:refnum<k35>)  [unwired: 7 in, 1 out]
      n226 = call "HoloLink_filter_features_by_frame.vi"("error in (no error)"=w412, "session in"=w413) -> ("error out"=w409:errorcluster, "Refnum out"=w410:refnum<k35>, "Frame"=w411:i32)  [unwired: 6 in, 1 out]
      n227 = call "HoloLink_filter_features_by_size.vi"("error in (no error)"=w409, "session in"=w410) -> ("error out"=w406:errorcluster, "return value"=w404:dbl[][], "Refnum out"=w405:refnum<k35>, "voxel_size"=w408:i32)  [unwired: 6 in]
      n228 = call "HoloLink_set_features.vi"("error in (no error)"=w406, "Features"=w404, "session in"=w405) -> ("error out"=w403:errorcluster, "Refnum out"=w402:refnum<k35>)  [unwired: 6 in, 1 out]
      n229 = call "HoloLink_link.vi"("error in (no error)"=w403, "session in"=w402) -> ("error out"=w398:errorcluster, "Refnum out"=w399:refnum<k35>, "memory"=w400:i32, "searchRange"=w401:T1)  [unwired: 5 in, 1 out]
      n230 = call "HoloLink_filter_trajectories_by_lenght.vi"("error in (no error)"=w398, "session in"=w399) -> ()  [unwired: 7 in, 3 out]
      n231 = call "HoloLink_get_one_trajectorie.vi"() -> ()  [unwired: 9 in, 3 out]
    }
    frame Enabled {
    }
  }
